vi "曾广骏ICRA2024最后的ratio控制.vi"() -> ()   [LabVIEW 2018]
doc: "Demonstrates the use of the Network Streams functions to send LED status to the myRIO target."
uses:
  <vilib>/ErrorRing/Error Ring.xnode
  <vilib>/vision/NI_Vision_Development_Module.lvlib
panel:
  out "期望ratio":dbl[](array[numeric])
  out "ratio误差的绝对值":dbl[](array[numeric])
  in  "pd":dbl=0.1
  out "最终的控制量":dbl
  in  "小p":dbl=2.0
  out "ratio误差的绝对值":dbl
  out "ratio的误差":dbl[](array[numeric])
  out "第二个前馈":dbl
  out "第一个前馈":dbl
  out "后一个ratio误差":dbl
  out "前一个ratio误差":dbl
  out "第一个i":i32
  out "第一次的predifined":dbl
  out "ratio的误差":dbl
  out "裁剪后的二值图":T1(plugin-control)
  in  "布尔":bool
  in  "ribbon磁场开关":bool=TRUE
  in  "期望ratio":dbl=5.0
  out "面积":sgl[](array[numeric])
  out "面积":sgl
  out "数据总":dbl[][](array[numeric])
  out "i":i32[](array[numeric])
  out "aspect ratio":dbl[](array[numeric])
  out "D2":i32[](array[numeric])
  out "D1":i32[](array[numeric])
  out "field ratio":sgl[](array[numeric])
  out "field ratio":sgl=4.0
  out "时间":i32
  in  "打开数据记录":bool
  out "aspect ratio":dbl
  out "D2":i32
  out "D1":i32
  out "二值图":T1(plugin-control)
  in  "Search Rect (entire image)":T2={"Left"=200, "Top"=120, "Right"=2000, "Bottom"=1920, "Rotation"=0.0} {"Rotation" format="%.2f"; "Left" scale=0.0..1024.0; "Right" scale=0.0..1024.0}
  out "备用的椭圆角度":sgl
  in  "Number of Erosion":i32=25
  out "Image 7":T1(plugin-control)
  in  "Acquisition Control::Acquisition Frame Rate":dbl=19.50304412841797 min=1.4211589097976685 max=44.94382095336914
  out "Stopped":bool
  in  "Stop (F) 2":bool caption="Stop (F)"
  out "Objects 2":T3(array[cluster]) {"Aspect Ratio" format="%.2f"; "Orientation" format="%.2f"; "Area" format="%.2f"; "Object Center"."Y" format="%.2f"; "Object Center"."X" format="%.2f"}
  in  "Settings 2":T4={"Objects"=0, "Threshold"=128, "Reject Border"=FALSE, "Fill Holes"=FALSE, "Min Object Size"=FALSE, "Min Size"=20000, "Max Object Size"=FALSE, "Max Size"=100, "Show Search Area"=FALSE, "Show Center"=TRUE, "Show Bounding Box"=TRUE} {"Objects" items=["Bright Objects", "Dark Objects"]; "Threshold" min=1 max=999999999 step=1; "Max Size" min=1 max=999999999 step=1; "Min Size" min=1 max=999999999 step=1}
  in  "Range 2":cluster{"Lower value":sgl, "Upper value":sgl}={"Lower value"=0.0, "Upper value"=230.0} {"Upper value" format="%.2f"; "Lower value" format="%.2f"}
  in  "Pause":bool
  out "Array":dbl[](array[numeric])
  in  "Parameter Settings":T5(tab)=enum."Ribbon Oscillating Field" caption="Field Types"
  in  "fg":dbl
  in  "pg":dbl
  in  "dg":dbl
  in  "Ag":dbl
  in  "AoOF":dbl
  in  "fo":sgl
  in  "do":sgl
  in  "oo":sgl
  in  "po":sgl
  in  "cc":sgl
  in  "pc":sgl
  in  "wc":sgl
  in  "dc":sgl
  in  "Ac":dbl
  in  "pr":sgl
  in  "Ar":dbl=8.0
  in  "wr":sgl=18.0
  in  "dr":sgl
  in  "Dis phase step":dbl
  in  "Dis phase frequency (Hz)":dbl
  in  "Dis tumbling frequency (Hz)":dbl
  in  "Dis strength(mT)":dbl
  in  "Swa strength (mT)":dbl
  in  "Swa frequency (Hz)":dbl
  in  "Swa pitch angle (deg)":dbl
  in  "Swa direction angle (deg)":dbl
  in  "Swa ratio":dbl=1.0
  in  "Pitch Angle (rotating around Constant, deg)":dbl
  in  "Ratio (A/C)":sgl=4.0
  in  "Direction Angle (deg)":sgl
  in  "Pitch Angle (rotating around Origin, deg)":sgl
  in  "Frequency (Hz)":sgl=10.0
  in  "Strength (mT)":dbl=10.0
  in  "Ar 2":dbl=5.0 caption="Ar"
  in  "ratio":sgl=1.0
  in  "运动方向":sgl
  in  "长轴方向":sgl
  in  "wr  2":sgl=8.0
  in  "速度大小":sgl
  out "Numeric 5":i32
  in  "Stop":bool
  out "error out":errorcluster
  in  "Target IP Address":string="172.22.11.2"
  # "Overview: Magnetic field calculation, and send parameters to myRIO\nInstructions:\n1. Verify the value of Target IP Address. Set Visa resource name.\n2. Ensure RT Main.vi is already running. \n3. Run this VI. Set parameters of magnetic field."
  # "Strength (mT)"
  # "Pitch Angle (deg)"
  # "Direction Angle (deg)"
  # "Frequency (Hz)"
  # "Strength (mT)"
  # "Oscilation Frequency (Hz)"
  # "Oscilation Angle (deg)"
  # "Pitch Angle (deg)"
  # "Direction Angle (deg)"
  # "Strength (mT)"
  # "Frequency (Hz)"
  # "Pitch Angle (deg)"
  # "Direction Angle (deg)"
  # "Conical Angle (deg)"
  # "Strength (mT)"
  # "Frequency (Hz)"
  # "Pitch Angle (deg)"
  # "Direction Angle (deg)"
  # "Strength (mT)"
  # "Tumbling Frequency (Hz)"
  # "Phase Frequency (Hz)"
  # "Phase Step"
  # "Strength (mT)"
  # "Frequency (Hz)"
  # "Pitch Angle (deg)"
  # "Direction Angle (deg)"
  # "Ratio"
  # "Strength (mT)"
  # "Frequency (Hz)"
  # "Ratio (A/C)"
  # "Direction Angle (deg)"
  # "Pitch Angle (rotating around Origin, deg)"
  # "Pitch Angle (rotating around Constant, deg)"
  # "Strength (mT)"
  # "Frequency (Hz)"
  # "Pitch Angle  (deg)"
  # "longaxis"
  # "Direction Angle (deg)"
  # "ratio (l/s)"
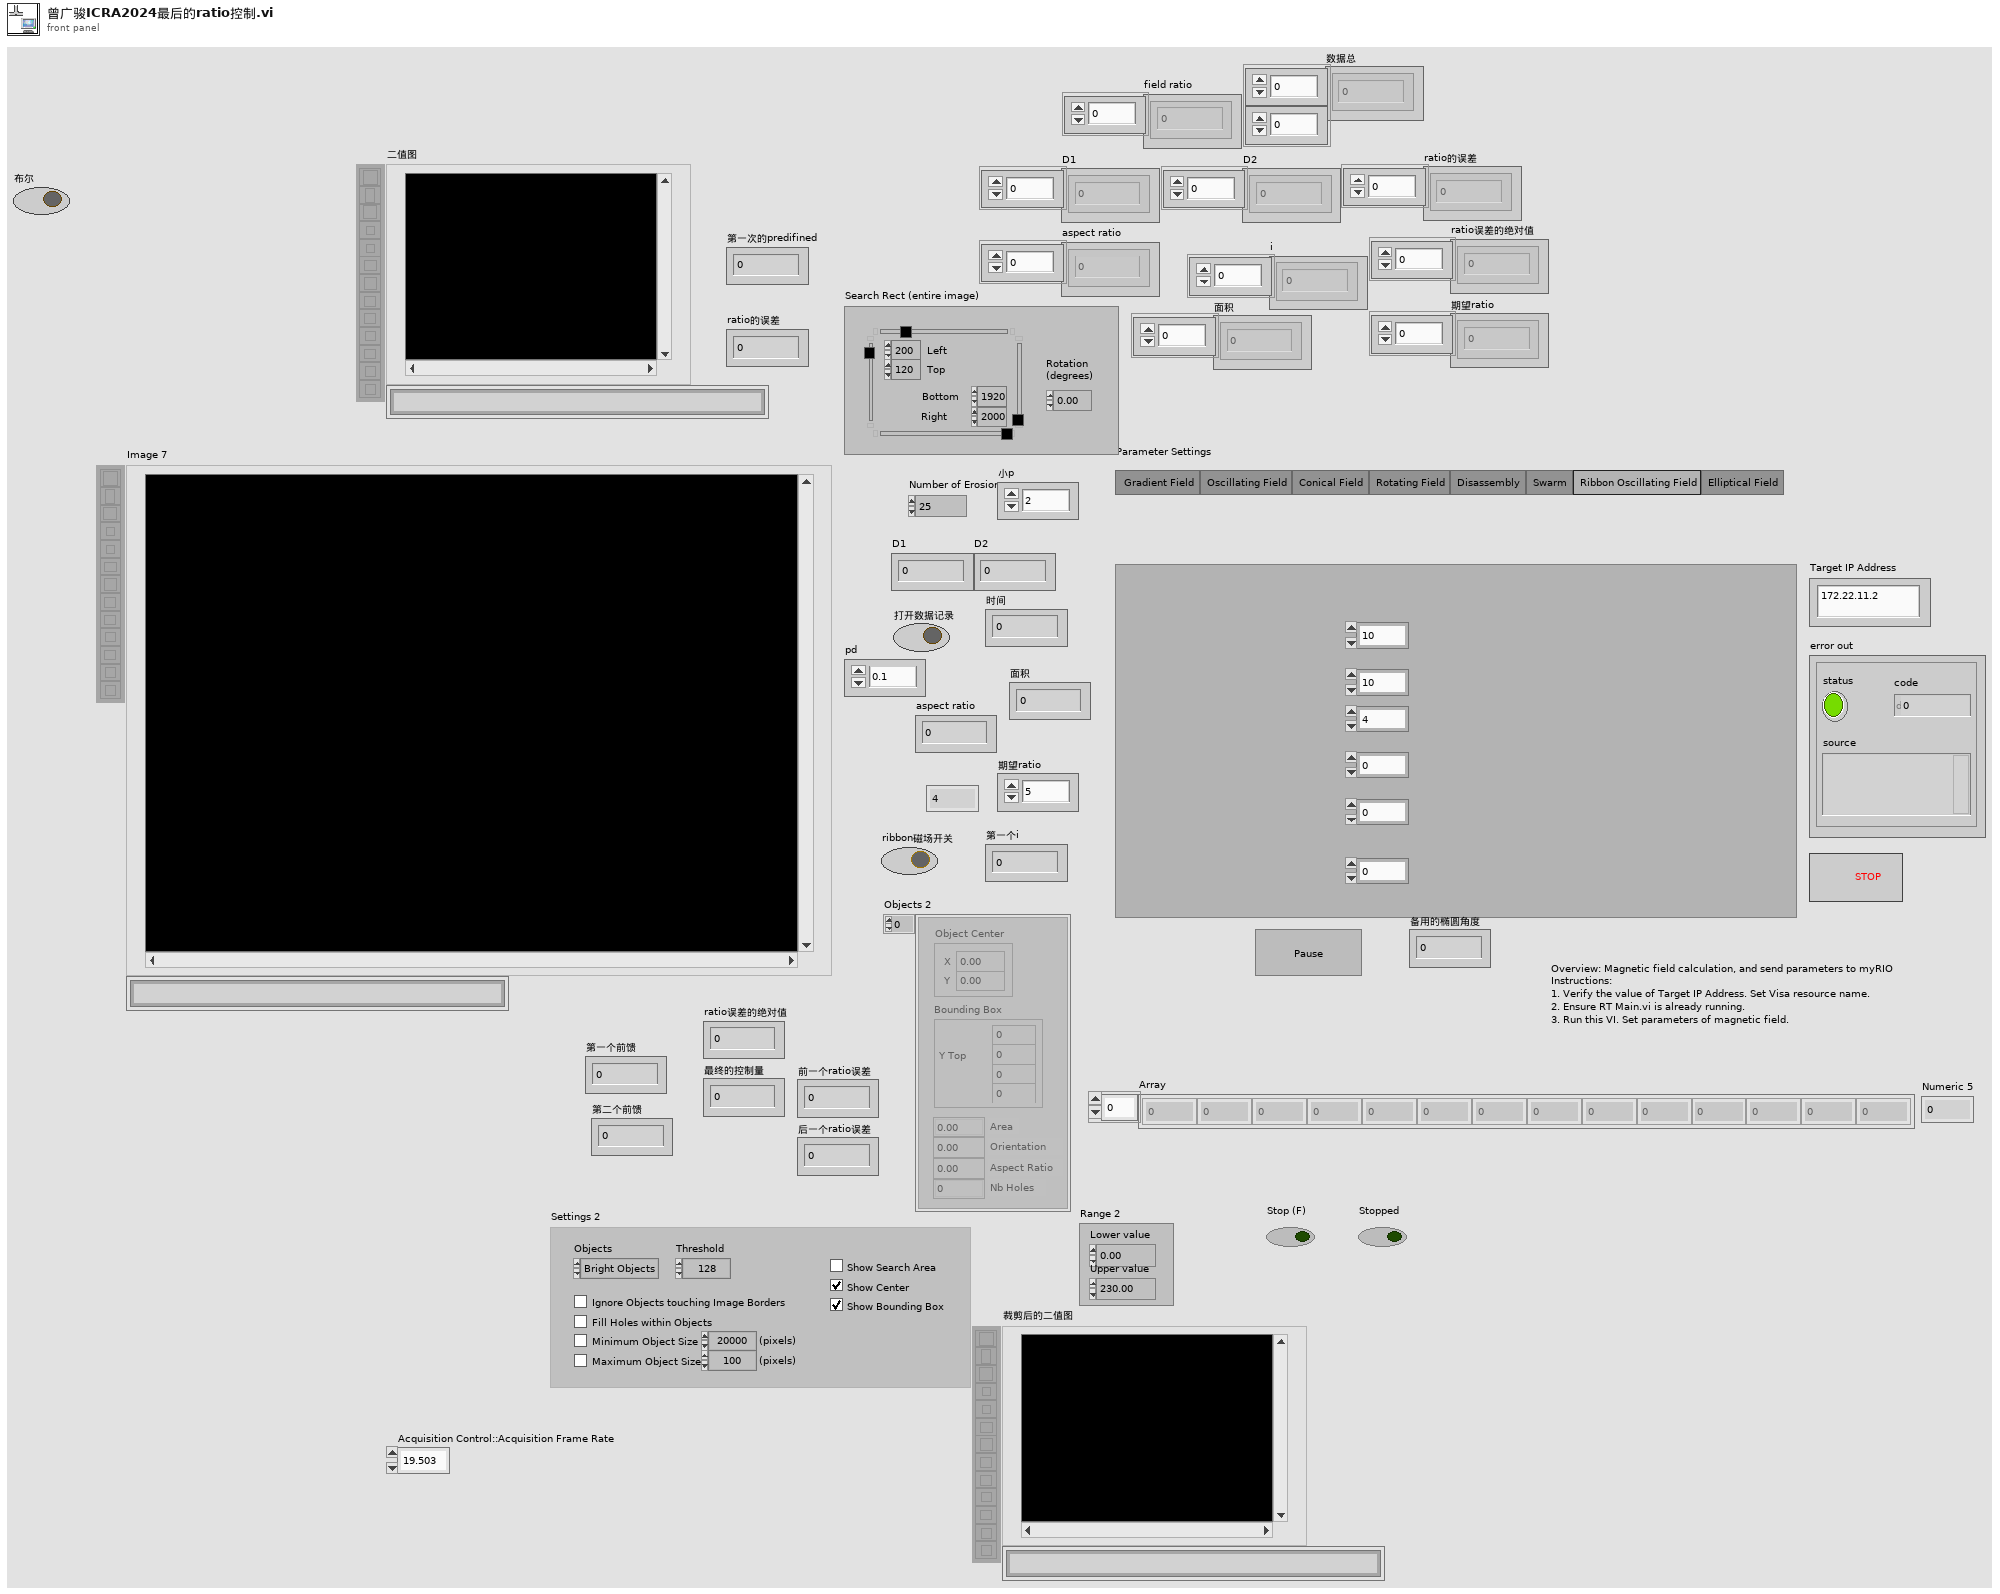
[diagram p1: front panel]
types:
  T1 = typedef "IMAQ Image.ctl" = refnum<image>
  T2 = typedef "IMAQ Rectangle" = cluster{"Left":i32, "Top":i32, "Right":i32, "Bottom":i32, "Rotation":dbl}
  T3 = cluster{"Object Center":cluster{"X":sgl, "Y":sgl}, "Bounding Box":cluster{"X Left":i32, "Y Top":i32, "X Right":i32, "Y Bottom":i32}, "Area":sgl, "Orientation":sgl, "Aspect Ratio":sgl, "Nb Holes":i32}[]
  T4 = cluster{"Objects":u16, "Threshold":i32, "Reject Border":bool, "Fill Holes":bool, "Min Object Size":bool, "Min Size":i32, "Max Object Size":bool, "Max Size":i32, "Show Search Area":bool, "Show Center":bool, "Show Bounding Box":bool}
  T5 = enum32{"Gradient Field ", "Oscillating Field", "Conical Field", "Rotating Field", "Disassembly", "Swarm", "Ribbon Oscillating Field", "Elliptical Field"}
  T6 = typedef "Image Type" = u32
  T7 = cluster{"Objects[0]":cluster{"Object Center":cluster{"X":sgl, "Y":sgl}, "Bounding Box":cluster{"X Left":i32, "Y Top":i32, "X Right":i32, "Y Bottom":i32}, "Area":sgl, "Orientation":sgl, "Aspect Ratio":sgl, "Nb Holes":i32}, "Objects[1]":cluster{"Object Center":cluster{"X":sgl, "Y":sgl}, "Bounding Box":cluster{"X Left":i32, "Y Top":i32, "X Right":i32, "Y Bottom":i32}, "Area":sgl, "Orientation":sgl, "Aspect Ratio":sgl, "Nb Holes":i32}, "Objects[2]":cluster{"Object Center":cluster{"X":sgl, "Y":sgl}, "Bounding Box":cluster{"X Left":i32, "Y Top":i32, "X Right":i32, "Y Bottom":i32}, "Area":sgl, "Orientation":sgl, "Aspect Ratio":sgl, "Nb Holes":i32}, "Objects[3]":cluster{"Object Center":cluster{"X":sgl, "Y":sgl}, "Bounding Box":cluster{"X Left":i32, "Y Top":i32, "X Right":i32, "Y Bottom":i32}, "Area":sgl, "Orientation":sgl, "Aspect Ratio":sgl, "Nb Holes":i32}, "Objects[4]":cluster{"Object Center":cluster{"X":sgl, "Y":sgl}, "Bounding Box":cluster{"X Left":i32, "Y Top":i32, "X Right":i32, "Y Bottom":i32}, "Area":sgl, "Orientation":sgl, "Aspect Ratio":sgl, "Nb Holes":i32}, "Objects[5]":cluster{"Object Center":cluster{"X":sgl, "Y":sgl}, "Bounding Box":cluster{"X Left":i32, "Y Top":i32, "X Right":i32, "Y Bottom":i32}, "Area":sgl, "Orientation":sgl, "Aspect Ratio":sgl, "Nb Holes":i32}, "Objects[6]":cluster{"Object Center":cluster{"X":sgl, "Y":sgl}, "Bounding Box":cluster{"X Left":i32, "Y Top":i32, "X Right":i32, "Y Bottom":i32}, "Area":sgl, "Orientation":sgl, "Aspect Ratio":sgl, "Nb Holes":i32}, "Objects[7]":cluster{"Object Center":cluster{"X":sgl, "Y":sgl}, "Bounding Box":cluster{"X Left":i32, "Y Top":i32, "X Right":i32, "Y Bottom":i32}, "Area":sgl, "Orientation":sgl, "Aspect Ratio":sgl, "Nb Holes":i32}, "Objects[8]":cluster{"Object Center":cluster{"X":sgl, "Y":sgl}, "Bounding Box":cluster{"X Left":i32, "Y Top":i32, "X Right":i32, "Y Bottom":i32}, "Area":sgl, "Orientation":sgl, "Aspect Ratio":sgl, "Nb Holes":i32}}
  T8 = cluster{"Object Center":cluster{"X":sgl, "Y":sgl}, "Bounding Box":cluster{"X Left":i32, "Y Top":i32, "X Right":i32, "Y Bottom":i32}, "Area":sgl, "Orientation":sgl, "Aspect Ratio":sgl, "Nb Holes":i32}
  T9 = cluster{"X Left":i32, "Y Top":i32, "X Right":i32, "Y Bottom":i32}
  T10 = typedef "ROI Descriptor" = cluster{"Global Rectangle":i32[], "Contours":cluster{"ID":enum32{"External", "Internal"}, "Type":u32, "Coordinates":i32[]}[]}
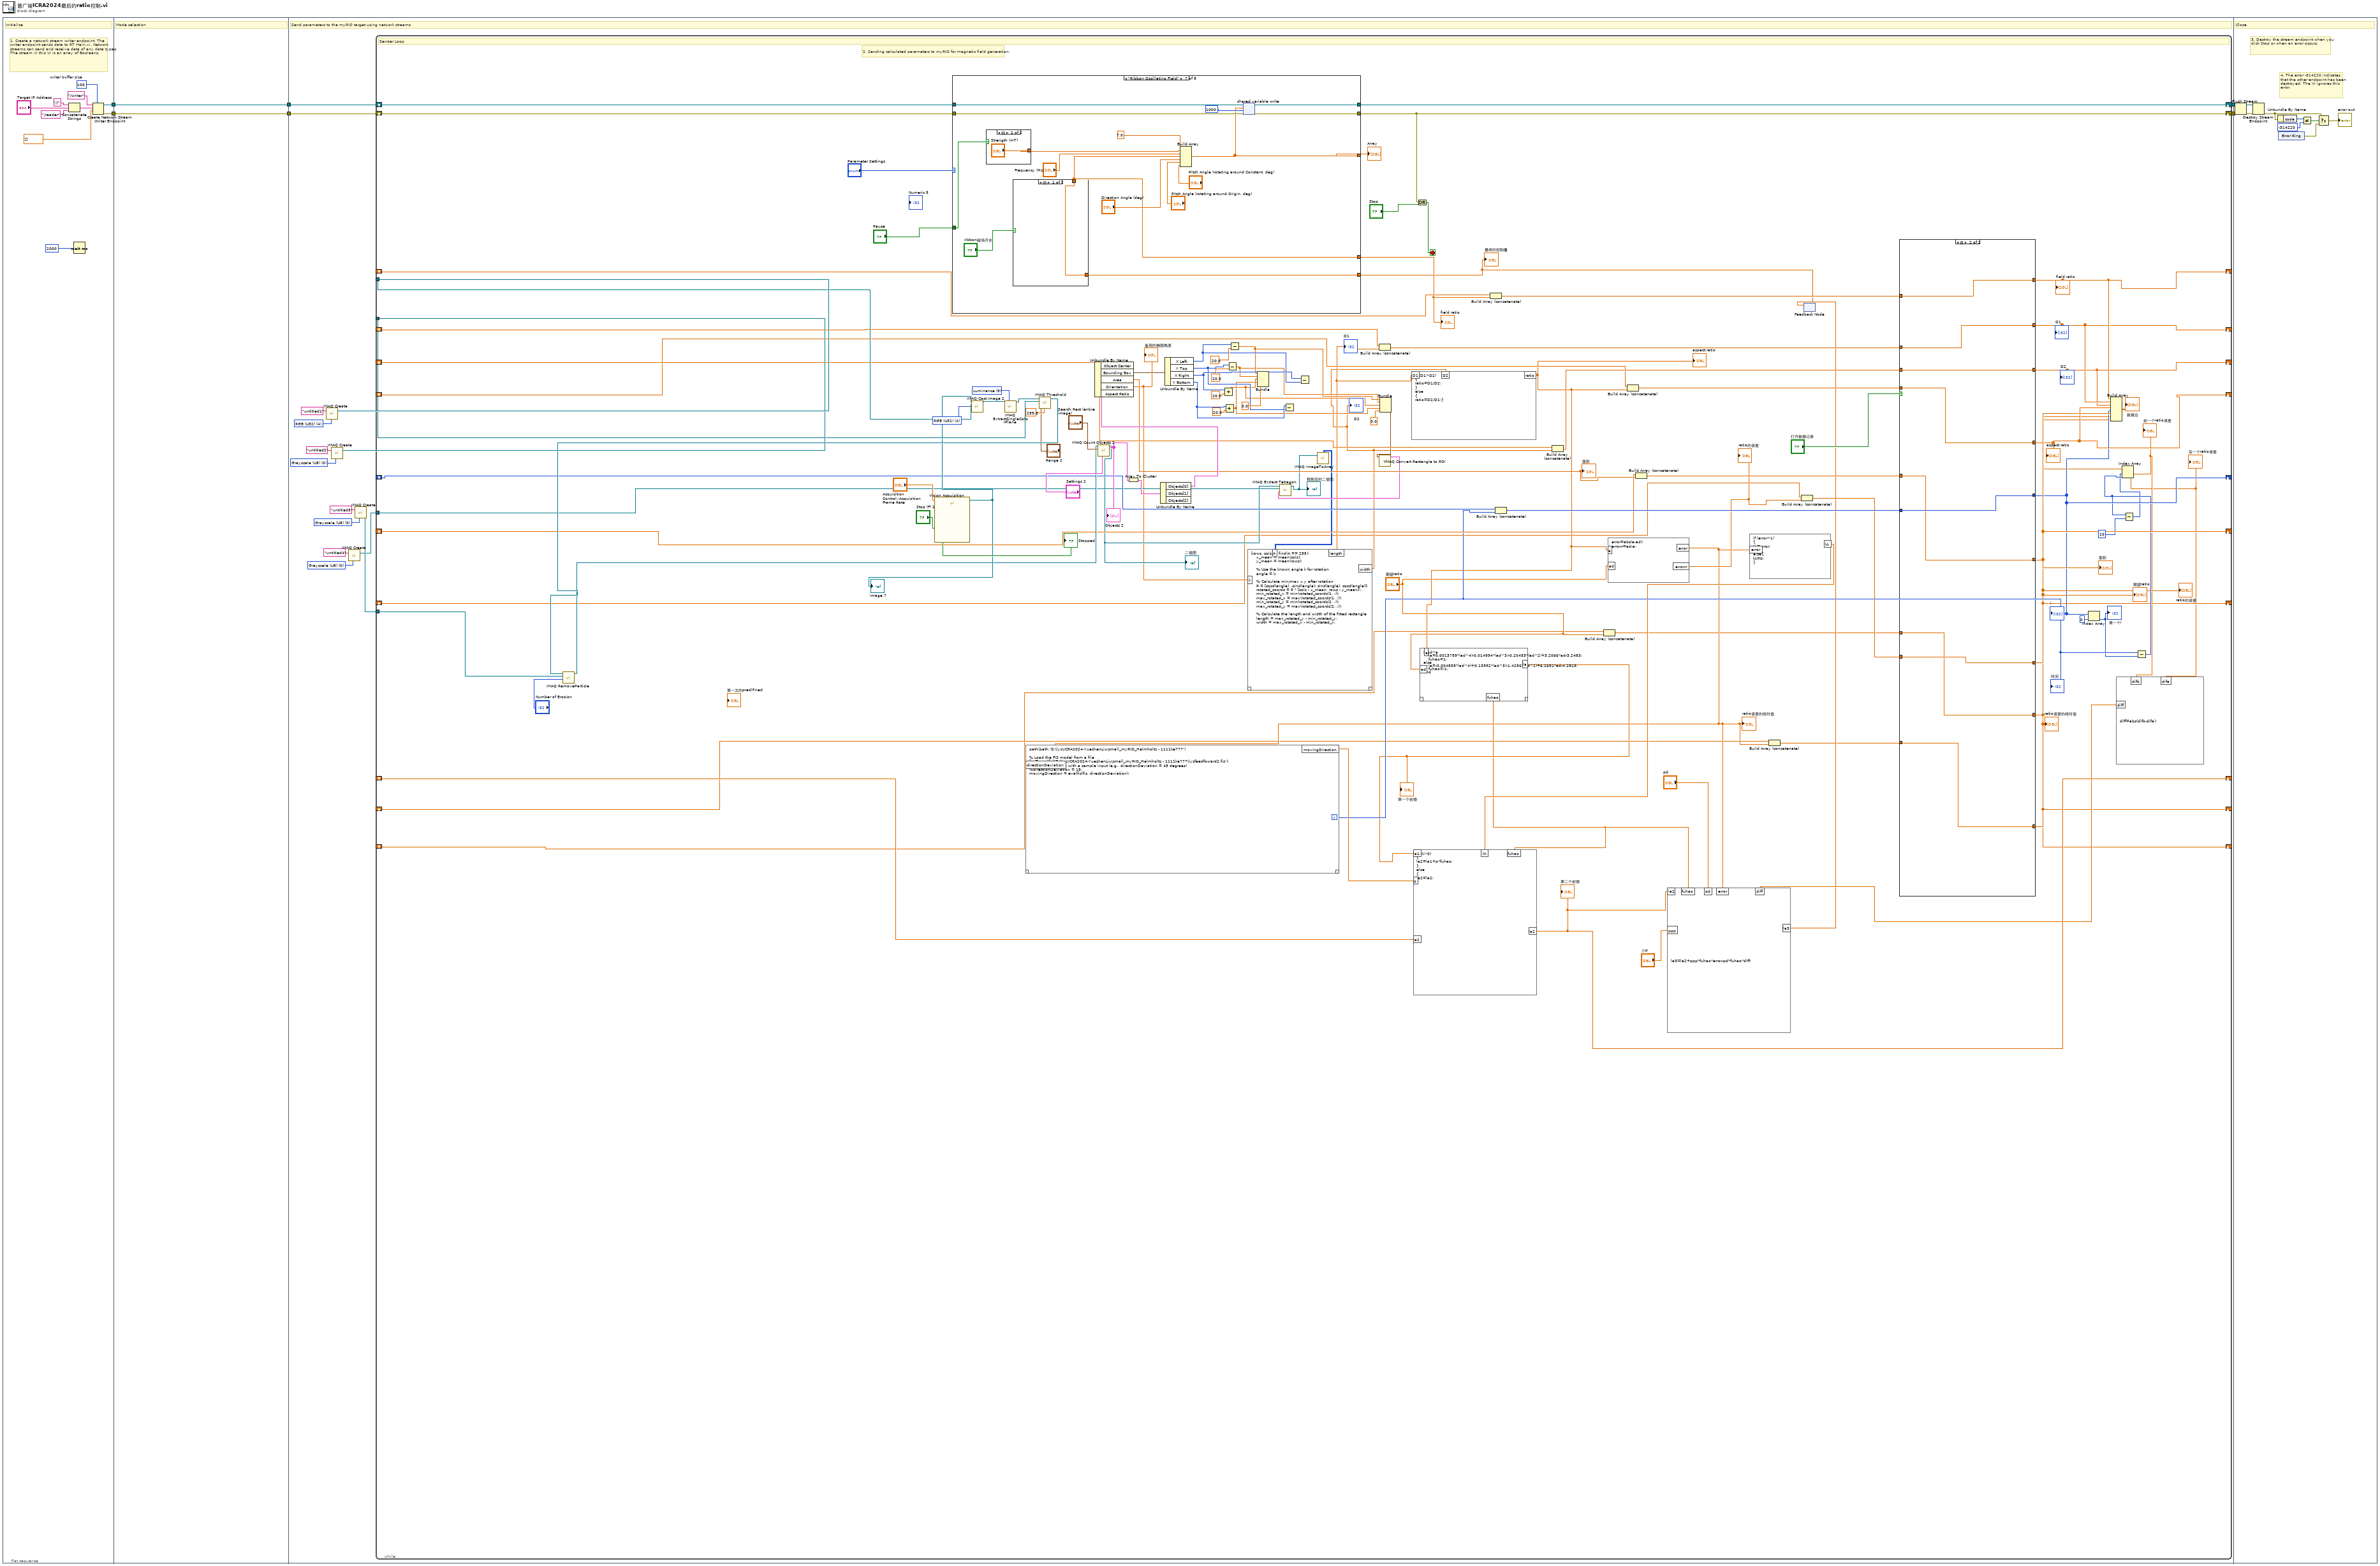
[diagram p0: block diagram]
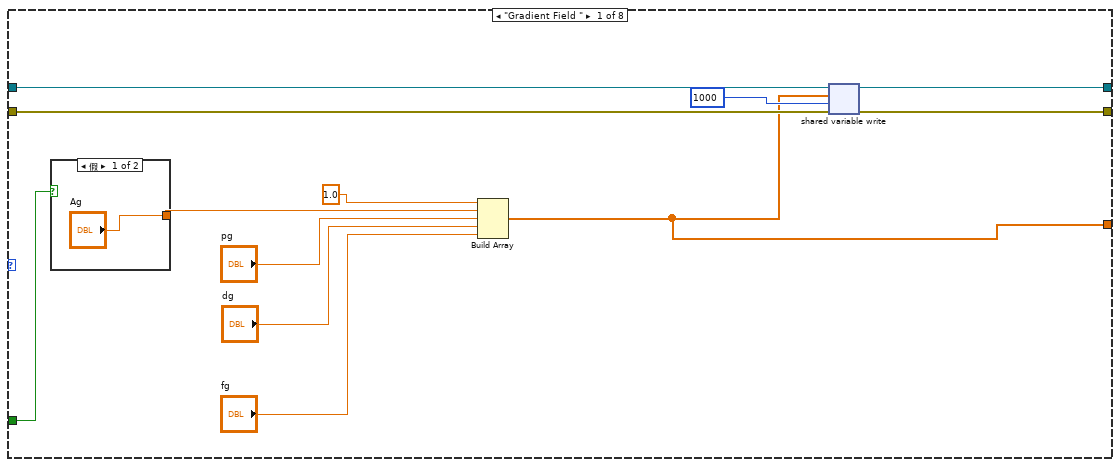
[diagram p3: hidden frame]
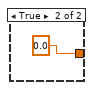
[diagram p4: hidden frame]
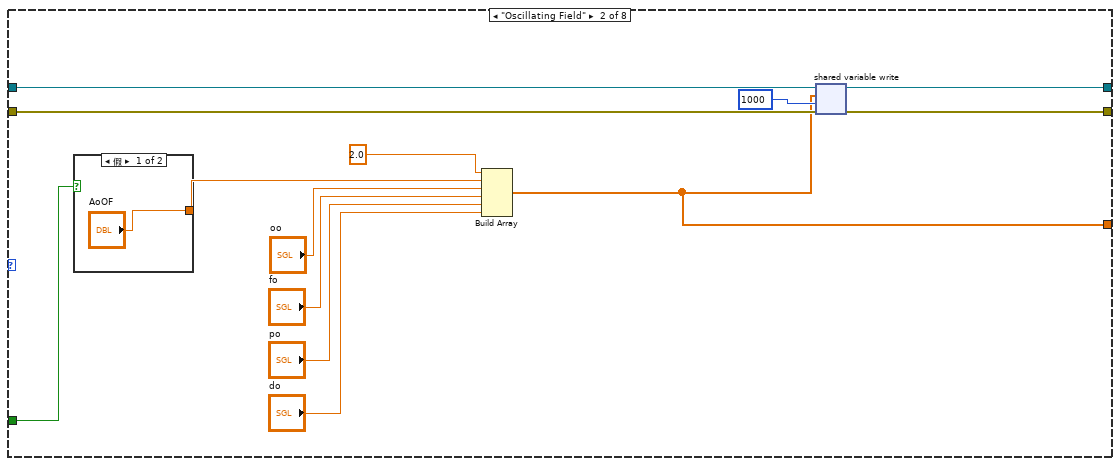
[diagram p5: hidden frame]
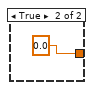
[diagram p6: hidden frame]
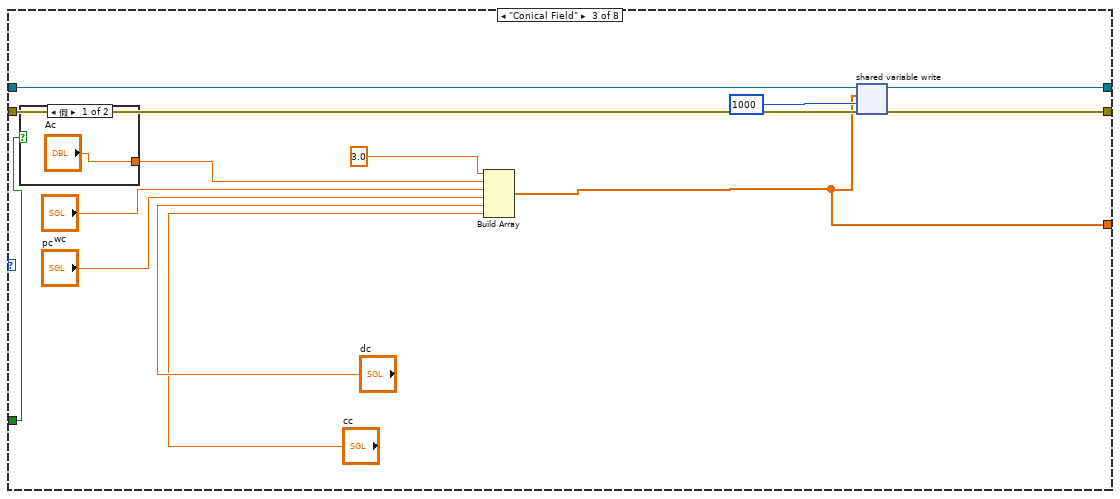
[diagram p7: hidden frame]
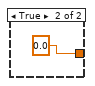
[diagram p8: hidden frame]
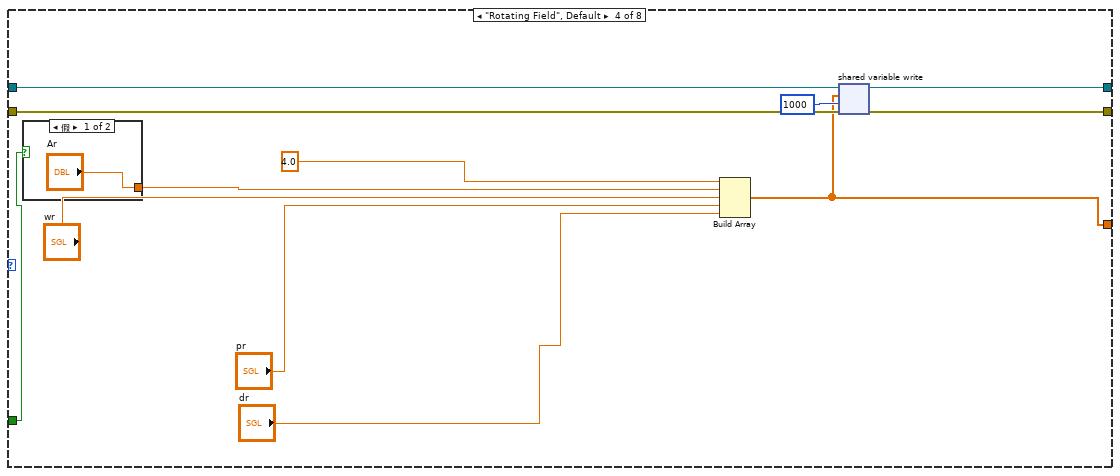
[diagram p9: hidden frame]
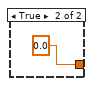
[diagram p10: hidden frame]
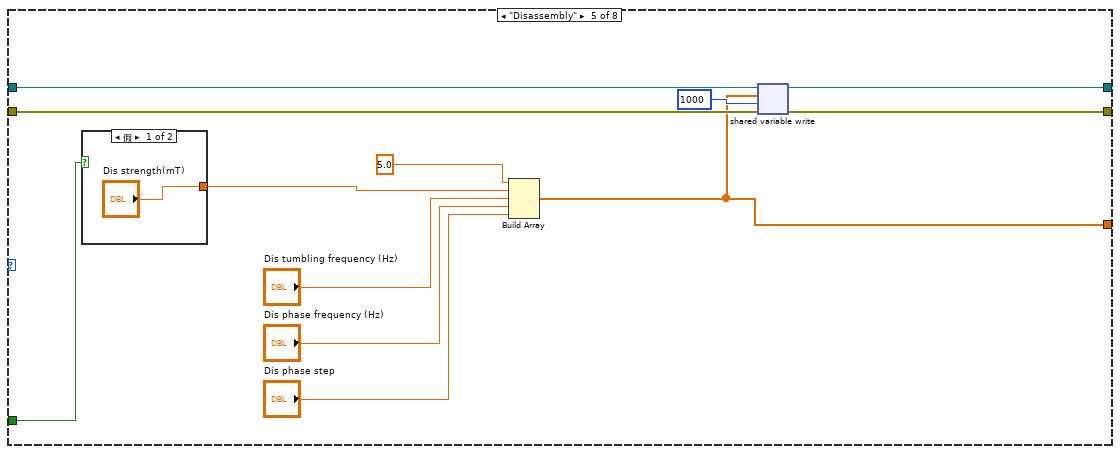
[diagram p11: hidden frame]
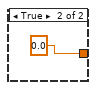
[diagram p12: hidden frame]
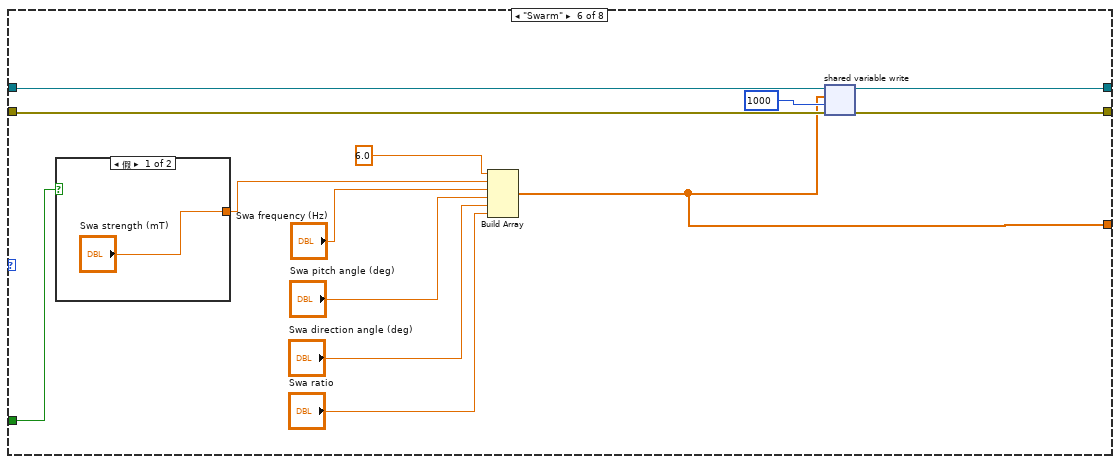
[diagram p13: hidden frame]
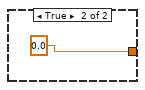
[diagram p14: hidden frame]
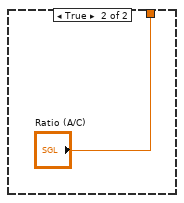
[diagram p15: hidden frame]
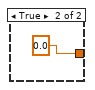
[diagram p16: hidden frame]
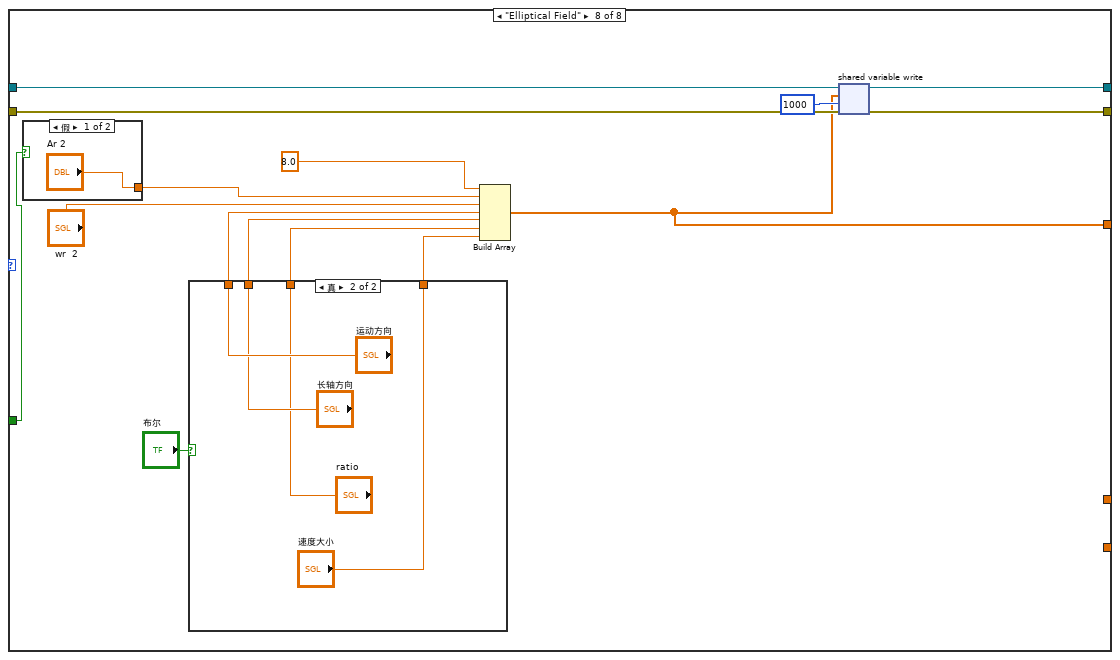
[diagram p17: hidden frame]
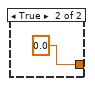
[diagram p19: hidden frame]
diagram:
  n1 = flat-sequence {
    tunnel: [w11] -> w2
    tunnel: [w10] -> w1
    tunnel: [w18] -> w4
    tunnel: [w17] -> w3
    tunnel: w1 -> [w17]
    tunnel: w2 -> [w18]
    tunnel: [w32] -> w6
    tunnel: w4 -> [w34]
    tunnel: [w31] -> w5
    tunnel: w3 -> [w33]
    tunnel: w6 -> [w289]
    tunnel: w5 -> [w286]
    frame #0 {
      w9 = 100  # writer buffer size
      # "1. Create a network stream writer endpoint. The writer endpoint sends data to RT Main.vi. Network streams can send and receive data of any data types. The stream in this VI is an array of Booleans."
      # "Initialize"
      n2 = Concatenate Strings("//", "Target IP Address", "/reader") -> (w16:string)
      n3 = Wait (ms)(milliseconds to wait=2000) -> ()  [unwired: 1 out]
      n4 = Create Network Stream Writer Endpoint(7:w9, 9:dbl[] [], 10:w16, 11:"/writer" ("reader name")) -> (0:w10:errorcluster, 3:w11:refnum<k21>)  [unwired: 3 in]
    }
    frame #1 {
      # "Mode selection"
    }
    frame #2 {
      w20 = T6 0 items=["Grayscale (U8)", "Grayscale (I16)", "Grayscale (SGL)", "Complex (CSG)", "RGB (U32)", "HSL (U32)", "RGB (U64)", "Grayscale (U16)"] ("Image Type")
      w23 = T6 0 items=["Grayscale (U8)", "Grayscale (I16)", "Grayscale (SGL)", "Complex (CSG)", "RGB (U32)", "HSL (U32)", "RGB (U64)", "Grayscale (U16)"] ("Image Type")
      w27 = T6 0 items=["Grayscale (U8)", "Grayscale (I16)", "Grayscale (SGL)", "Complex (CSG)", "RGB (U32)", "HSL (U32)", "RGB (U64)", "Grayscale (U16)"] ("Image Type")
      w29 = T6 4 items=["Grayscale (U8)", "Grayscale (I16)", "Grayscale (SGL)", "Complex (CSG)", "RGB (U32)", "HSL (U32)", "RGB (U64)", "Grayscale (U16)"] ("Image Type")
      # "Send parameters to the myRIO target using network streams"
      n5 = call "IMAQ Create"("Image Name"="untitled1", "Image Type"=w29) -> ("New Image"=w26:T1)  [unwired: 3 in, 1 out]
      n6 = call "IMAQ Create"("Image Name"="untitled2", "Image Type"=w27) -> ("New Image"=w25:T1)  [unwired: 3 in, 1 out]
      n7 = call "IMAQ Create"("Image Name"="untitled4", "Image Type"=w20) -> ("New Image"=w19:T1)  [unwired: 3 in, 1 out]
      n8 = call "IMAQ Create"("Image Name"="untitled3", "Image Type"=w23) -> ("New Image"=w22:T1)  [unwired: 3 in, 1 out]
      n9 = while {
        shift-right: [w138] -> w31
        shift-left: w33 -> [w140]
        shift-right: [w139] -> w32
        shift-left: w34 -> [w141]
        tunnel: w25 -> [w129]
        tunnel: w26 -> [w124]
        tunnel: w22 -> [w113]
        shift-right: [w90] -> _
        shift-left: _ -> [w99]
        shift-right: [w89] -> _
        shift-left: _ -> [w97]
        shift-right: [w88] -> _
        shift-left: _ -> [w95]
        shift-right: [w69] -> _
        shift-left: _ -> [w93]
        shift-right: [w68] -> _
        shift-left: _ -> [w91]
        shift-right: [w84] -> _
        shift-left: _ -> [w83]
        tunnel: w19 -> [w82]
        shift-right: [w58] -> _
        shift-left: _ -> [w59]
        shift-right: [w56] -> _
        shift-left: _ -> [w55]
        shift-right: [w39] -> _
        shift-left: _ -> [w40]
        shift-right: [w35] -> _
        shift-left: _ -> [w36]
        i -> [w66]
        stop <- w128 stop-if-true
        w123 = T6 4 items=["Grayscale (U8)", "Grayscale (I16)", "Grayscale (SGL)", "Complex (CSG)", "RGB (U32)", "HSL (U32)", "RGB (U64)", "Grayscale (U16)"] ("Image Type")
        w134 = 5 items=["Red", "Green", "Blue", "Hue", "Saturation", "Luminance", "Value", "Intensity"] ("Color Plane")
        # "2. Sending calculated parameters to myRIO for magnetic field generation."
        # "Sender Loop"
        n10 = call "Vision Acquisition"("Acquisition Control::Acquisition Frame Rate"="Acquisition Control::Acquisition Frame Rate", "Stop (F)"="Stop (F) 2") -> ("Image Out"=w106:T1, "Stopped"=→"Stopped":bool)  [unwired: 23 in, 1 out]
        "Image 7" <- w106
        n11 = call "IMAQ Cast Image 2"("Image Src"=w106, "Image Dst"=w124, "Image Type"=w123) -> ("Image Dst Out"=w125:T1)  [unwired: 11 in, 1 out]
        n12 = call "IMAQ ExtractSingleColorPlane"("Color Plane"=w134, "Image Src"=w125) -> ("Image Dst Out"=w111:T1)  [unwired: 8 in, 1 out]
        n13 = call "IMAQ Threshold"("Replace Value"=sgl 255.0, "Range"="Range 2", "Image Dst"=w129, "Image Src"=w111) -> ("Image Dst Out"=w114:T1)  [unwired: 6 in, 1 out]
        n14 = call "IMAQ RemoveParticle"("Number of Erosion"="Number of Erosion", "Image Dst"=w113, "Image Src"=w114) -> ("Image Dst Out"=w105:T1)  [unwired: 7 in, 1 out]
        n15 = call "IMAQ Count Objects 2"("Settings"="Settings 2", "Search Rect (entire image)"="Search Rect (entire image)", "Image"=w105) -> ("Image Out"=w81:T1, "Objects"=w130:T3)  [unwired: 4 in, 3 out]
        "Objects 2" <- w130
        "二值图" <- w81
        n16 = Array To Cluster(array=w130) -> (cluster=w116:T7)
        n17 = Unbundle By Name(w116) -> ("Objects[0]"=w115:T8)  [unwired: 2 out]
        n18 = Unbundle By Name(w115) -> ("Bounding Box"=w122:T9, "Area"=w86:sgl, "Orientation"=w64:sgl)  [unwired: 2 out]
        "备用的椭圆角度" <- w64
        "面积" <- w86
        n19 = Unbundle By Name(w122) -> ("X Left"=w108:i32, "Y Top"=w103:i32, "X Right"=w109:i32, "Y Bottom"=w104:i32)
        n20 = Add(x=w109, y=20.0) -> (x+y=w76:dbl)
        n21 = Add(x=w104, y=20.0) -> (x+y=w75:dbl)
        n22 = Subtract(x=w103, y=20.0) -> (x-y=w77:dbl)
        n23 = Subtract(x=w108, y=20.0) -> (x-y=w78:dbl)
        n24 = Bundle(w78, w77, w76, w75, 0.0) -> ()  [unwired: 1 in, 1 out]
        n25 = Subtract(x=w104, y=w103) -> ()  [unwired: 1 out]
        n26 = Subtract(x=w109, y=w108) -> ()  [unwired: 1 out]
        n27 = Bundle(w78, w77, w76, w75, 0.0) -> (w73:cluster{dbl, dbl, dbl, dbl, dbl})  [unwired: 1 in]
        n28 = call "IMAQ Convert Rectangle to ROI"("Rectangle"=w73) -> ("ROI Descriptor"=w79:T10)  [unwired: 8 in, 1 out]
        n29 = call-poly "IMAQ Extract Tetragon"("ROI Descriptor"=w79, "Image Dst"=w82, "Image Src"=w81) -> ("Image Dst Out"=w80:T1)  [unwired: 7 in, 1 out]
        "裁剪后的二值图" <- w80
        n30 = call "IMAQ ImageToArray"("Image"=w80) -> ("Image Pixels (U8)"=w72:u8[][])  [unwired: 3 in, 4 out]
        n31 = script code="[rows, cols] = find(A == 255);\n    x_mean = mean(cols);\n    y_mean = mean(rows);\n\n    % Use the known angle k for rotation\n    angle = k;\n\n    % Calculate min/max x,y after rotation\n    R = [cosd(angle), -sind(angle); sind(angle), cosd(angle)];\n    rotated_coords = R * [cols - x_mean, rows - y_mean]';\n    min_rotated_x = min(rotated_coords(1, :));\n    max_rotated_x = max(rotated_coords(1, :));\n    min_rotated_y = min(rotated_coords(2, :));\n    max_rotated_y = max(rotated_coords(2, :));\n\n    % Calculate the length and width of the fitted rectangle\n    length = max_rotated_y - min_rotated_y;\n    width = max_rotated_x - min_rotated_x;"("A"=w72, "k"=w64) -> ("length"=w71:dbl, "width"=w70:dbl)  [unwired: 1 in, 1 out]
        "D1" <- w71
        "D2" <- w70
        n32 = Build Array (concatenate)(w97, w71) -> (w98:dbl[])
        n33 = formula code="if (D1>D2)\n{\nratio=D1/D2;\n}\nelse\n{\nratio=D2/D1;}"("D1"=w71, "D2"=w70) -> ("ratio"=w44:dbl)
        "aspect ratio" <- w44
        n34 = script code="if ad>a\n    la=0.0013759*(ad^4)-0.014994*(ad^3)-0.20453*(ad^2)+3.2066*ad-3.2483;\n    fuhao=1;\nelse\n    la=-0.004839*(ad^4)+0.13992*(ad^3)-1.4256*(ad^2)+6.2651*ad-4.2815;\n    fuhao=-1;\nend"("a"=w44, "ad"="期望ratio") -> ("la"=w46:dbl, "fuhao"=w45:dbl)  [unwired: 1 in, 1 out]
        "第一个前馈" <- w46
        n35 = Build Array (concatenate)(w91, w66) -> (w92:i32[])
        n36 = Build Array (concatenate)(w95, w70) -> (w96:dbl[])
        n37 = Build Array (concatenate)(w36, "期望ratio") -> (w37:dbl[])
        n38 = formula code="error=abs(a-ad);\nerrorrr=ad-a;"("a"=w44, "ad"="期望ratio") -> ("error"=w42:dbl, "errorrr"=w51:dbl)
        "ratio的误差" <- w51
        "ratio误差的绝对值" <- w42
        n39 = script code="path(path,'D:\\lyz\\ICRA2024-YuezhenLiu\\small_myRIO_Helmholtz - 1111ke777')\n\n% Load the FIS model from a file\nfis = readfis('D:\\lyz\\ICRA2024-YuezhenLiu\\small_myRIO_Helmholtz - 1111ke777\\lyzfeedfoward2.fis');\n% Evaluate the FIS with a sample input (e.g., directionDeviation = 45 degrees)\n%directionDeviation = 15;\nmovingDirection = evalfis(fis, directionDeviation);"("directionDeviation"=w42) -> ("movingDirection"=w43:dbl)  [unwired: 1 in, 1 out]
        n40 = Build Array (concatenate)(w93, w44) -> (w94:dbl[])
        n41 = Build Array (concatenate)(w83, w86) -> (w85:sgl[])
        n42 = formula code="if (error>1)\n{\nkk=error;\n}\nelse{\nkk=0;\n}"("error"=w42) -> ("kk"=w60:dbl)
        n43 = formula code="if(kk>0)\n{\nla2=la1+p*fuhao;\n}\nelse\n{\nla2=la2;\n}"("kk"=w60, "la1"=w46, "fuhao"=w45, "p"=w43, "la2"=w59) -> ("la2"=w58:dbl)
        "第二个前馈" <- w58
        n44 = Build Array (concatenate)(w40, w42) -> (w41:dbl[])
        n45 = Build Array (concatenate)(w55, w51) -> (w57:dbl[])
        n46 = feedback #1() -> (w48:dbl)  [unwired: 1 in]
        "最终的控制量" <- w48
        n47 = case shown="\"Ribbon Oscillating Field\"" "Parameter Settings" {
          tunnel: w141 -> [w162 w177 w192 w206 w220 w234 w254 w272]
          tunnel: w140 -> [w159 w176 w191 w205 w218 w233 w252 w271]
          tunnel: [w161 w175 w189 w204 w219 w232 w253 w270] -> w139
          tunnel: [w160 w174 w190 w203 w217 w231 w251 w269] -> w138
          tunnel: [w155 w168 w183 w198 w211 w226 w249 w264] -> w137
          tunnel: "Pause" -> [w153 w166 w181 w196 w210 w225 w245 w262]
          tunnel: [_ _ _ _ _ _ w242 _] -> w101
          tunnel: w48 -> [_ _ _ _ _ _ w239 _]
          frame "Gradient Field " {
            n48 = case shown="假" w153 {
              tunnel: ["Ag" 0.0] -> w154
              frame False {
              }
              frame True {
              }
            }
            n49 = Build Array(1.0, w154, "pg", "dg", "fg") -> (w155:dbl[])
            n50 = shared-variable-write(w162, w159, w155, 1000 ("timeout ms (-1)")) -> (w161:refnum<k21>, w160:errorcluster)  [unwired: 1 out]
          }
          frame "Oscillating Field" {
            n51 = case shown="假" w166 {
              tunnel: ["AoOF" 0.0] -> w167
              frame False {
              }
              frame True {
              }
            }
            n52 = Build Array(2.0, w167, "oo", "fo", "po", "do") -> (w168:dbl[])
            n53 = shared-variable-write(w177, w176, w168, 1000 ("timeout ms (-1)")) -> (w175:refnum<k21>, w174:errorcluster)  [unwired: 1 out]
          }
          frame "Conical Field" {
            # "FG"
            n54 = case shown="假" w181 {
              tunnel: ["Ac" 0.0] -> w182
              frame False {
              }
              frame True {
              }
            }
            n55 = Build Array(3.0, w182, "wc", "pc", "dc", "cc") -> (w183:dbl[])
            n56 = shared-variable-write(w192, w191, w183, 1000 ("timeout ms (-1)")) -> (w189:refnum<k21>, w190:errorcluster)  [unwired: 1 out]
          }
          frame "Rotating Field", Default {
            n57 = case shown="假" w196 {
              tunnel: ["Ar" 0.0] -> w197
              frame False {
              }
              frame True {
              }
            }
            n58 = Build Array(4.0, w197, "wr", "pr", "dr") -> (w198:dbl[])
            n59 = shared-variable-write(w206, w205, w198, 1000 ("timeout ms (-1)")) -> (w204:refnum<k21>, w203:errorcluster)  [unwired: 1 out]
          }
          frame "Disassembly" {
            n60 = case shown="假" w210 {
              tunnel: ["Dis strength(mT)" 0.0] -> w215
              frame False {
              }
              frame True {
              }
            }
            n61 = Build Array(5.0, w215, "Dis tumbling frequency (Hz)", "Dis phase frequency (Hz)", "Dis phase step") -> (w211:dbl[])
            n62 = shared-variable-write(w220, w218, w211, 1000 ("timeout ms (-1)")) -> (w219:refnum<k21>, w217:errorcluster)  [unwired: 1 out]
          }
          frame "Swarm" {
            n63 = case shown="假" w225 {
              tunnel: ["Swa strength (mT)" 0.0] -> w224
              frame False {
              }
              frame True {
              }
            }
            n64 = Build Array(6.0, w224, "Swa frequency (Hz)", "Swa pitch angle (deg)", "Swa direction angle (deg)", "Swa ratio") -> (w226:dbl[])
            n65 = shared-variable-write(w234, w233, w226, 1000 ("timeout ms (-1)")) -> (w232:refnum<k21>, w231:errorcluster)  [unwired: 1 out]
          }
          frame "Ribbon Oscillating Field" {
            n66 = case shown="假" w245 {
              tunnel: ["Strength (mT)" 0.0] -> w244
              frame False {
              }
              frame True {
              }
            }
            n67 = case shown="假" "ribbon磁场开关" {
              tunnel: [w255 "Ratio (A/C)"] -> w242
              tunnel: w239 -> [w255 _]
              frame False {
              }
              frame True {
              }
            }
            n68 = Build Array(7.0, w244, "Frequency (Hz)", w242, "Direction Angle (deg)", "Pitch Angle (rotating around Origin, deg)", "Pitch Angle (rotating around Constant, deg)") -> (w249:dbl[])
            n69 = shared-variable-write(w254, w252, w249, 1000 ("timeout ms (-1)")) -> (w253:refnum<k21>, w251:errorcluster)  [unwired: 1 out]
          }
          frame "Elliptical Field" {
            n70 = case shown="假" w262 {
              tunnel: ["Ar 2" 0.0] -> w263
              frame False {
              }
              frame True {
              }
            }
            n71 = case shown="真" "布尔" {
              tunnel: [_ "运动方向"] -> w267
              tunnel: [_ "长轴方向"] -> w266
              tunnel: [_ "ratio"] -> w261
              tunnel: [_ "速度大小"] -> w260
              frame False {
              }
              frame True {
              }
            }
            n72 = Build Array(8.0, w263, "wr  2", w267, w266, w261, w260) -> (w264:dbl[])
            n73 = shared-variable-write(w272, w271, w264, 1000 ("timeout ms (-1)")) -> (w270:refnum<k21>, w269:errorcluster)  [unwired: 1 out]
          }
        }
        "Array" <- w137
        "field ratio" <- w101
        n74 = Or(x=w138, y="Stop") -> (x .or. y?=w128:bool)
        n75 = Build Array (concatenate)(w99, w101) -> (w100:dbl[])
        n76 = case shown="真" "打开数据记录" {
          tunnel: [_ w151] -> w90
          tunnel: w100 -> [_ w151]
          tunnel: [_ w150] -> w89
          tunnel: w98 -> [_ w150]
          tunnel: [_ w149] -> w88
          tunnel: w96 -> [_ w149]
          tunnel: [_ w148] -> w69
          tunnel: w94 -> [_ w148]
          tunnel: [_ w147] -> w68
          tunnel: w92 -> [_ w147]
          tunnel: [_ w146] -> w84
          tunnel: w85 -> [_ w146]
          tunnel: [_ w145] -> w56
          tunnel: w57 -> [_ w145]
          tunnel: [_ w144] -> w39
          tunnel: w41 -> [_ w144]
          tunnel: [_ w143] -> w35
          tunnel: w37 -> [_ w143]
          frame False {
          }
          frame True {
          }
        }
        "field ratio" <- w90
        "D1" <- w89
        "D2" <- w88
        "aspect ratio" <- w69
        "i" <- w68
        "面积" <- w84
        "ratio的误差" <- w56
        "ratio误差的绝对值" <- w39
        "期望ratio" <- w35
        n77 = Index Array(array=w68, index=0 ("索引")) -> (element=w65:i32)
        "第一个i" <- w65
        n78 = Build Array(w90, w89, w88, w69, w68, w84, w39, w35) -> (→"数据总":dbl[][])
        n79 = Subtract(x=w66, y=w65) -> (x-y=w63:i32)
        n80 = Subtract(x=w63, y=10) -> (x-y=w62:i32)
        n81 = Index Array(array=w56, index #1=w62, index #2=w63) -> (element #1=w54:dbl, element #2=w53:dbl)
        "前一个ratio误差" <- w54
        "后一个ratio误差" <- w53
        n82 = formula code="diff=abs(difb-difa);"("difb"=w54, "difa"=w53) -> ("diff"=w52:dbl)
        n83 = formula code="la3=la2+ppp*fuhao*error-pd*fuhao*diff;"("la2"=w58, "fuhao"=w45, "diff"=w52, "ppp"="小p", "pd"="pd", "error"=w42) -> ("la3"=w49:dbl)
        n84 = feedback-in #1(w49) -> ()
        "时间" <- w66
      }
    }
    frame #3 {
      # "4. The error -314220 indicates that the other endpoint has been destroyed. The VI ignores this error."
      # "3. Destroy the stream endpoint when you click Stop or when an error occurs."
      # "Close"
      n85 = Flush Stream(8:w286, 11:w289) -> (0:w287:errorcluster, 3:w288:refnum<k21>)  [unwired: 2 in, 1 out]
      n86 = Destroy Stream Endpoint(8:w287, 11:w288) -> (0:w281:errorcluster)
      n87 = Unbundle By Name(w281) -> ("code"=w285:i32)
      n88 = xnode "Error Ring"() -> ("错误输出"=w282:errorcluster)
      n89 = Not Equal?(x=w285, y=-314220) -> (x != y?=w283:bool)
      n90 = Select(t=w281, s=w283, f=w282) -> (s? t:f=→"error out":errorcluster)
    }
  }
